vi "Fpga-MicroBlaze-Receive.vi"(0 "niInstr Network API FPGA v1.lvclass":refnum<class "niInstr Network API FPGA v1.lvclass">, 1 "Port RX Clear Counts":bool, 2 "RX FIFO":refnum<k21>) -> (4 "debug data":T1)   [LabVIEW 2017, in "My Network FPGA v1.lvlib"]
uses:
  Example SubVIs/My Network FPGA v1.lvlib
  <instrlib>/_niInstr/Network/API/v1/FPGA/niInstr Network API FPGA v1.lvclass
  <instrlib>/_niInstr/Network/Ethernet/MAC/Data Stream/v1/Read Data Stream.vi
  <instrlib>/_niInstr/Network/Ethernet/MAC/Data Stream/v1/Read End of Good Frame.vi
  <instrlib>/_niInstr/Basic Elements/v1/FPGA/Private/Count Up U32.vi
  <instrlib>/_niInstr/Network/Ethernet/MAC/Data Stream/v1/Read End of Bad Frame.vi
  <vilib>/rvi/DataTransferAndStorage/Container/Common/niFpgaContainerExecOnDevCompGetState.vi
  <vilib>/rvi/Emulation/niFpgaSctlEmulationGetInTimedLoop.vi
  <vilib>/rvi/errors/niFpgaSetErrorForExecOnDevCompSimple.vi
  <vilib>/rvi/eio/common/nirviEmuReportErrorAndStop.vi
  <vilib>/rvi/interface/RandomDataEmulation/nirviRandomDataAcquireLock.vi
  <vilib>/rvi/interface/RandomDataEmulation/nirviRandomDataQueueStore.vi
  <vilib>/rvi/interface/RandomDataEmulation/nirviRandomDataReleaseLock.vi
  <vilib>/rvi/interface/RandomDataEmulation/nirviFPGAContextMergeError.vi
  <vilib>/rvi/interface/RandomDataEmulation/nirviRandomDataCheckExitLoopConditions.vi
  <vilib>/express/rvi/timingcommon/nirviCommon.vi
  <vilib>/rvi/interface/RandomDataEmulation/niFpgaRandomDataHandleErrors.vi
  <vilib>/rvi/DataTransferAndStorage/Container/XNode/niFpgaContainer.xnode
  <vilib>/rvi/FIFO/Fifo_Resource/niFpgaFifoEmulationRefInMultiElement.vi
  <instrlib>/_niInstr/Network/Ethernet/MAC/Data Stream/v1/niInstr Ethernet MAC Data Stream v1.lvclass
  <instrlib>/_niInstr/Basic Elements/v1/FPGA/niInstr Basic Elements v1 FPGA.lvlib
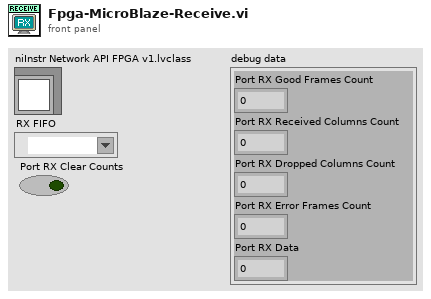
[diagram p1: front panel]
types:
  T1 = cluster{"Port RX Good Frames Count":u32, "Port RX Received Columns Count":u32, "Port RX Dropped Columns Count":u32, "Port RX Error Frames Count":u32, "Port RX Data":u64}
  T2 = typedef "niInstr Ethernet Utilities FPGA v1.lvlib/Network Data Stream.ctl" = cluster{"data":u8[], "data valid":bool, "byte enables":bool[]}
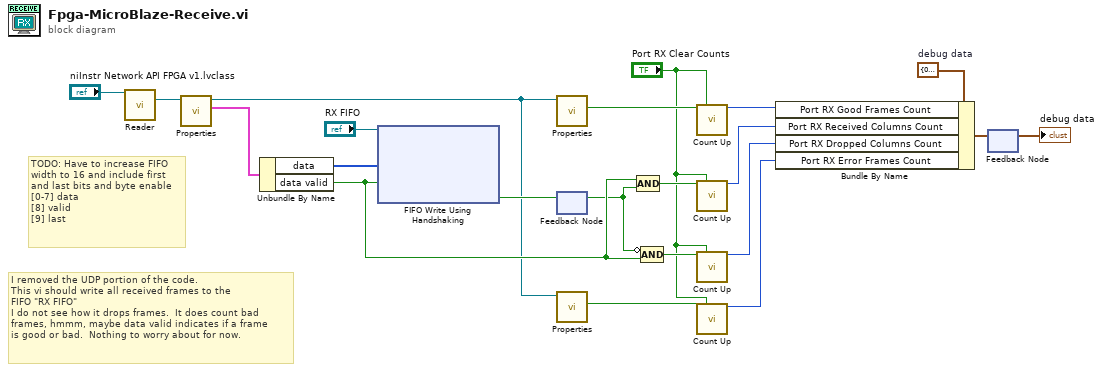
[diagram p0: block diagram]
diagram:
  w20 = T1 {"Port RX Good Frames Count"=0, "Port RX Received Columns Count"=0, "Port RX Dropped Columns Count"=0, "Port RX Error Frames Count"=0, "Port RX Data"=0}  # debug data
  # "TODO: Have to increase FIFO\nwidth to 16 and include first\nand last bits and byte enable\n[0-7] data\n[8] valid\n[9] last"
  # "I removed the UDP portion of the code.\nThis vi should write all received frames to the \nFIFO \"RX FIFO\"\nI do not see how it drops frames.  It does count bad\nframes, hmmm, maybe data valid indicates if a frame\nis good or bad.  Nothing to worry about for now."
  n1 = call <instrlib>:"Reader.vi"("niInstr Network API FPGA v1.lvclass"="niInstr Network API FPGA v1.lvclass") -> ("niInstr Ethernet MAC Data Stream v1 out"=w2:refnum<class "niInstr Ethernet MAC Data Stream v1.lvclass">)  [unwired: 13 in, 1 out]
  n2 = call-poly <instrlib>:"Properties.vi"("niInstr Ethernet MAC Data Stream v1 in"=w2) -> ("Data Stream"=w1:T2, "niInstr Ethernet MAC Data Stream v1 out"=w3:refnum<class "niInstr Ethernet MAC Data Stream v1.lvclass">)  [unwired: 9 in]
  n3 = Unbundle By Name(w1) -> ("data"=w18:u8[], "data valid"=w17:bool)
  n4 = xnode ("FIFO Write Using Handshaking")("Element"=w18, "Input Valid"=w17, "FIFO In"="RX FIFO") -> ("Ready for Input"=w16:bool)  [unwired: 1 out]
  n5 = call-poly <instrlib>:"Properties.vi"("niInstr Ethernet MAC Data Stream v1 in"=w3) -> ("End of Good Frame"=w14:bool)  [unwired: 9 in, 1 out]
  n6 = feedback #1() -> (w15:bool)  [unwired: 1 in]
  n7 = feedback-in #1(w16) -> ()
  n8 = call-poly <instrlib>:"Properties.vi"("niInstr Ethernet MAC Data Stream v1 in"=w3) -> ("End of Bad Frame"=w8:bool)  [unwired: 9 in, 1 out]
  n9 = Compound Arithmetic op=AND(w17, w15) -> (w12:bool)
  n10 = Compound Arithmetic op=AND(invert w15, w17) -> (w10:bool)
  n11 = call-poly <instrlib>:"Count Up.vi"("increment"=w14, "reset"="Port RX Clear Counts") -> ("count out"=w13:u32)  [unwired: 13 in]
  n12 = call-poly <instrlib>:"Count Up.vi"("increment"=w12, "reset"="Port RX Clear Counts") -> ("count out"=w11:u32)  [unwired: 13 in]
  n13 = call-poly <instrlib>:"Count Up.vi"("increment"=w10, "reset"="Port RX Clear Counts") -> ("count out"=w9:u32)  [unwired: 13 in]
  n14 = call-poly <instrlib>:"Count Up.vi"("increment"=w8, "reset"="Port RX Clear Counts") -> ("count out"=w7:u32)  [unwired: 13 in]
  n15 = Bundle By Name(cluster=w20, "Port RX Good Frames Count"=w13, "Port RX Received Columns Count"=w11, "Port RX Dropped Columns Count"=w9, "Port RX Error Frames Count"=w7) -> (w21:T1)
  n16 = feedback-in #2(w21) -> ()
  n17 = feedback #2() -> (→"debug data":T1)  [unwired: 1 in]
